vi "Calculate surface gradient of Gamma.vi"(1 "Panel linked to E2":T1={"V0"=[], "V1"=[], "V2"=[], "E0"=[], "E1"=[], "E2"=[], "n^"=[], "Pc"=[], "Gamma'"=0.0, "V_transp."=0.0, "E0 link"=-1, "E1 link"=-1, "E2 link"=-1}, 2 "Panel linked to E1":T1={"V0"=[], "V1"=[], "V2"=[], "E0"=[], "E1"=[], "E2"=[], "n^"=[], "Pc"=[], "Gamma'"=0.0, "V_transp."=0.0, "E0 link"=-1, "E1 link"=-1, "E2 link"=-1}, 3 "Panel linked to E0":T1={"V0"=[], "V1"=[], "V2"=[], "E0"=[], "E1"=[], "E2"=[], "n^"=[], "Pc"=[], "Gamma'"=0.0, "V_transp."=0.0, "E0 link"=-1, "E1 link"=-1, "E2 link"=-1}, 4 "Centre panel n^":sgl[](array[numeric])) -> (0 "0.5*Grad_s(Gamma)":sgl[](array[numeric]))   [LabVIEW 2017]
uses:
  ctls/Triangle panel.ctl
panel:
  # "PN 24/10/17"
  # "Vertices"
  # "Edges"
  # "Unit normal"
  # "Control point"
  # "Edge\nlinks \n(tri index)"
  # "Vertices"
  # "Edges"
  # "Unit normal"
  # "Control point"
  # "Edge\nlinks \n(tri index)"
  # "Vertices"
  # "Edges"
  # "Unit normal"
  # "Control point"
  # "Edge\nlinks \n(tri index)"
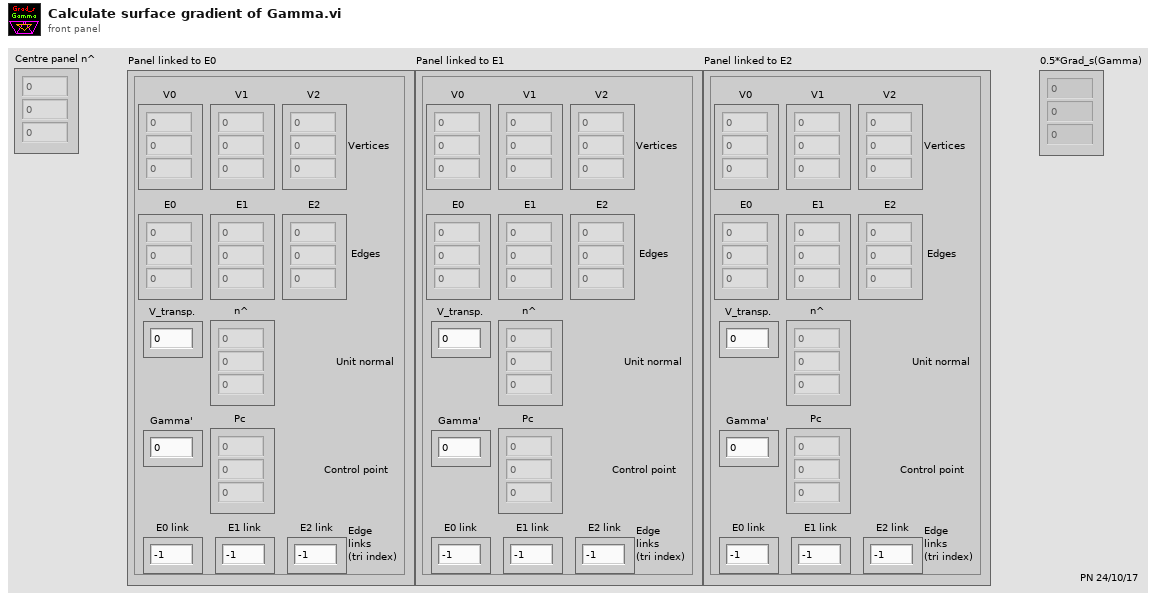
[diagram p1: front panel]
types:
  T1 = typedef "Triangle panel.ctl" = cluster{"V0":sgl[], "V1":sgl[], "V2":sgl[], "E0":sgl[], "E1":sgl[], "E2":sgl[], "n^":sgl[], "Pc":sgl[], "Gamma'":sgl, "V_transp.":sgl, "E0 link":i32, "E1 link":i32, "E2 link":i32}
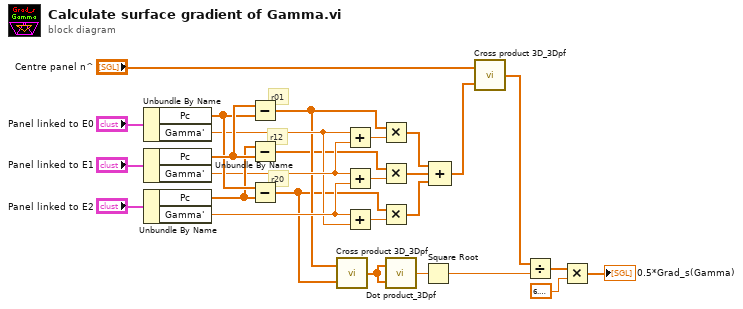
[diagram p0: block diagram]
diagram:
  # "r20"
  # "r12"
  # "r01"
  n1 = Unbundle By Name("Panel linked to E0") -> ("Pc"=w23:sgl[], "Gamma'"=w15:sgl)
  n2 = Unbundle By Name("Panel linked to E1") -> ("Pc"=w24:sgl[], "Gamma'"=w17:sgl)
  n3 = Unbundle By Name("Panel linked to E2") -> ("Pc"=w22:sgl[], "Gamma'"=w16:sgl)
  n4 = Subtract(x=w24, y=w23) -> (x-y=w13:sgl[])
  n5 = Subtract(x=w22, y=w24) -> (x-y=w11:sgl[])
  n6 = Subtract(x=w23, y=w22) -> (x-y=w9:sgl[])
  n7 = call "Cross product 3D_3Dpf.vi"("B"=w9, "A"=w13) -> ("A x B"=w19:sgl[])
  n8 = Add(x=w15, y=w17) -> (x+y=w14:sgl)
  n9 = Add(x=w17, y=w16) -> (x+y=w12:sgl)
  n10 = Add(x=w16, y=w15) -> (x+y=w10:sgl)
  n11 = Multiply(x=w13, y=w14) -> (x*y=w8:sgl[])
  n12 = Multiply(x=w11, y=w12) -> (x*y=w7:sgl[])
  n13 = Multiply(x=w9, y=w10) -> (x*y=w6:sgl[])
  n14 = call "Dot product_3Dpf.vi"("B"=w19, "A"=w19) -> ("A . B"=w20:sgl)
  n15 = Square Root(x=w20) -> (sqrt(x)=w4:sgl)
  n16 = Compound Arithmetic op=ADD(w8, w7, w6) -> (w5:sgl[])
  n17 = call "Cross product 3D_3Dpf.vi"("B"=w5, "A"="Centre panel n^") -> ("A x B"=w21:sgl[])
  n18 = Divide(x=w21, y=w4) -> (x/y=w3:sgl[])
  n19 = Multiply(x=w3, y=sgl 6.2831855) -> (x*y=→"0.5*Grad_s(Gamma)":sgl[])
